vi "New Case tester.vi"() -> ()   [LabVIEW 2020, in "Method Generation.lvlib" / "Getter Generator.lvclass"]
uses:
  Getter Generator.lvclass
  Getter Generator.lvclass/Getter Generator.ctl
panel:
  in  "error in (no error)":errorcluster
  out "error out":errorcluster
  out "output cluster":refnum<class "Getter Generator.lvclass">
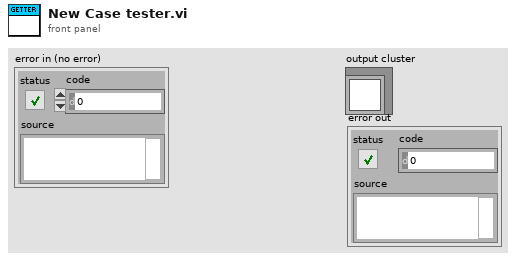
[diagram p1: front panel]
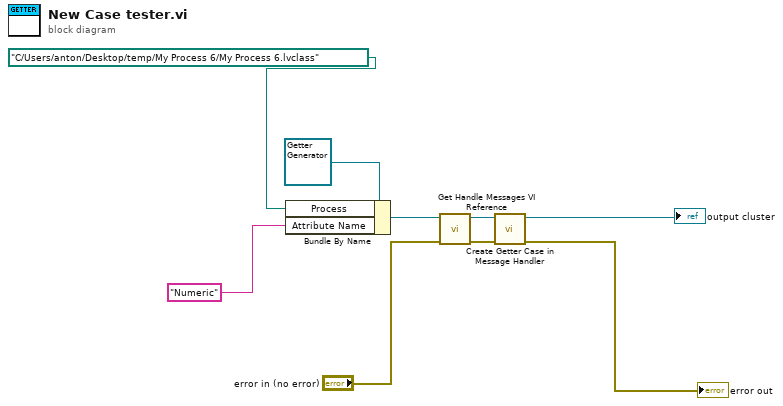
[diagram p0: block diagram]
diagram:
  n1 = Bundle By Name(cluster=refnum<class "Getter Generator.lvclass"> refnum ("New Getter Dialog In"), "Process"=path "C:/Users/anton/Desktop/temp/My Process 6/My Process 6.lvclass" ("class path"), "Attribute Name"="Numeric") -> (w7:refnum<class "Getter Generator.lvclass">)
  n2 = call "Get Handle Messages VI Reference.vi"("error in (no error)"="error in (no error)", "Getter Generator in"=w7) -> ("error out"=w2:errorcluster, "Getter Generator out"=w5:refnum<class "Getter Generator.lvclass">)  [unwired: 8 in]
  n3 = call "Create Getter Case in Message Handler.vi"("error in (no error)"=w2, "Getter Generator in"=w5) -> ("error out"=→"error out":errorcluster, "Getter Generator out"=→"output cluster":refnum<class "Getter Generator.lvclass">)  [unwired: 8 in]
